vi "create.vi"(8 "error in (no error)":errorcluster, 9 "handle":i32, 10 "client":i32) -> (0 "error out":errorcluster, 3 "VideoCreateStaging out":refnum<class "VideoCreateStaging.lvclass">)   [LabVIEW 2020, in "VideoCreateStaging.lvclass"]
uses:
  VideoCreateStaging.lvclass
  VideoCreateStaging.lvclass/VideoCreateStaging.ctl
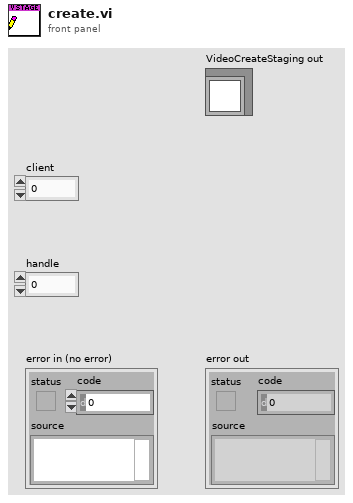
[diagram p1: front panel]
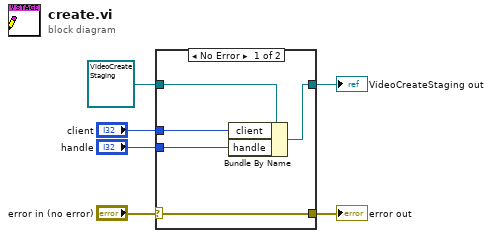
[diagram p0: block diagram]
diagram:
  n1 = case shown="No Error" "error in (no error)" {
    selector: "error in (no error)" -> [w11 w12]
    tunnel: [w11 w12] -> w5
    tunnel: [w9 w13] -> w3
    tunnel: refnum<class "VideoCreateStaging.lvclass"> refnum ("VideoCreateStaging in") -> [w10 w13]
    tunnel: "client" -> [w8 _]
    tunnel: "handle" -> [w7 _]
    frame No Error {
      n2 = Bundle By Name(cluster=w10, "client"=w8, "handle"=w7) -> (w9:refnum<class "VideoCreateStaging.lvclass">)
    }
    frame Error {
    }
  }
  "error out" <- w5
  "VideoCreateStaging out" <- w3
